vi "ValueSignalByName.vi"(0 "VI Reference In":refnum<vi>, 2 "delimiter (>>)":string=">>", 5 "Control Name":string, 7 "Value (Signaling)":variant, 11 "error in":errorcluster) -> (4 "VI Reference Out":refnum<vi>, 15 "error out":errorcluster)   [LabVIEW 2016]
doc: "This VI sets the value of top level controls in other VI"
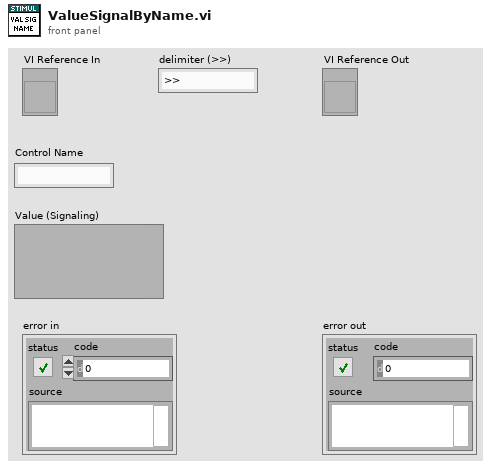
[diagram p1: front panel]
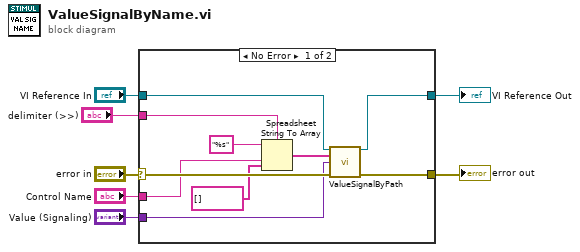
[diagram p0: block diagram]
diagram:
  n1 = case shown="No Error" "error in" {
    selector: "error in" -> [w17 w19]
    tunnel: "Control Name" -> [w12 _]
    tunnel: "VI Reference In" -> [w14 w18]
    tunnel: [w13 w18] -> w4
    tunnel: "Value (Signaling)" -> [w15 _]
    tunnel: [w16 w19] -> w2
    tunnel: "delimiter (>>)" -> [w8 _]
    frame No Error {
      n2 = Spreadsheet String To Array(delimiter (Tab)=w8, format string="%s", spreadsheet string=w12, array type (2D Dbl)=string[] []) -> (array=w10:string[])
      n3 = call "ValueSignalByPath.vi"("VI Reference In"=w14, "Control Path"=w10, "Value (Signaling)"=w15, "error in"=w17) -> ("VI Reference Out"=w13:refnum<vi>, "error out"=w16:errorcluster)  [unwired: 10 in]
    }
    frame Error {
    }
  }
  "error out" <- w2
  "VI Reference Out" <- w4
